vi "Configure Setpoints Range Limits.vi"(7 "Unit Address (1)":u8=1, 8 "error in (no error)":errorcluster, 9 "Range Limit Value (0)":i32, 10 "Limit Type (False)":bool, 11 "VISA resource name":refnum<visa-resource-name>) -> (0 "error out":errorcluster, 3 "VISA resource name out":refnum<visa-resource-name>)   [LabVIEW 2014, in "Eurotherm 35xx Series.lvlib"]
doc: "This VI sets the Range limits of Setpoints.\n\nWarning: This VI uses Controller Configuration Mode, this interrupts working process (device will not control).\nIt is recommended that the device should be disconnected from any active process."
uses:
  <instrlib>/Eurotherm 35xx Series/Eurotherm 35xx Series.lvlib
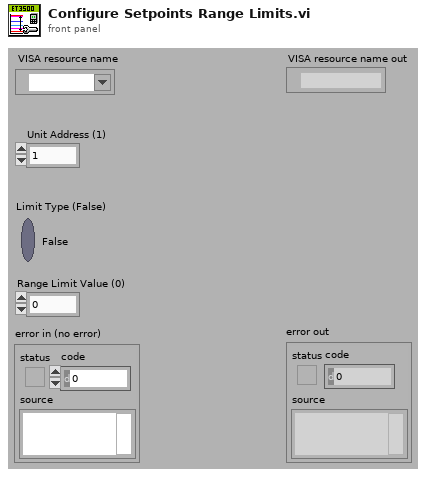
[diagram p1: front panel]
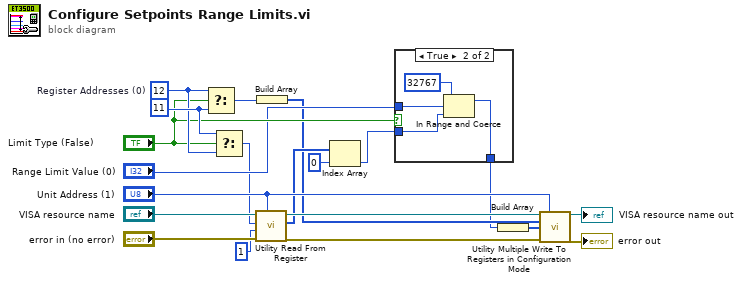
[diagram p0: block diagram]
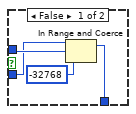
[diagram p2: hidden frame]
diagram:
  w12 = 11 ("Register Addresses (0)")
  w11 = 12  # Register Addresses (0)
  n1 = Select(t=w11, s="Limit Type (False)", f=w12) -> (s? t:f=w4:i32)
  n2 = Select(t=w12, s="Limit Type (False)", f=w11) -> (s? t:f=w5:i32)
  n3 = call <instrlib>:"Utility Read From Register.vi"("Unit Address (1)"="Unit Address (1)", "error in (no error)"="error in (no error)", "Num Of Reg (1)"=u16 1, "Register Address (0)"=w5, "VISA resource name"="VISA resource name") -> ("error out"=w16:errorcluster, "Data"=w10:i16[], "VISA resource name out"=w17:refnum<visa-resource-name>)  [unwired: 4 in]
  n4 = Build Array(w4) -> (w3:i32[])
  n5 = Index Array(array=w10, index=0) -> (element=w7:i16)
  n6 = case shown="True" "Limit Type (False)" {
    tunnel: w7 -> [w22 w27]
    tunnel: "Range Limit Value (0)" -> [w24 w26]
    tunnel: [w21 w25] -> w1
    frame False {
      n7 = In Range and Coerce(upper limit=w22, x=w24, lower limit=-32768 ("upper limit")) -> (coerced(x)=w21:i32)  [unwired: 1 out]
    }
    frame True {
      n8 = In Range and Coerce(upper limit=32767, x=w26, lower limit=w27) -> (coerced(x)=w25:i32)  [unwired: 1 out]
    }
  }
  n9 = Build Array(w1) -> (w2:i32[])
  n10 = call <instrlib>:"Utility Multiple Write To Registers in Configuration Mode.vi"("VISA resource name"=w17, "Unit Address (1)"="Unit Address (1)", "Registers Addresses (0)"=w3, "Data (0)"=w2, "error in (no error)"=w16) -> ("VISA resource name out"=→"VISA resource name out":refnum<visa-resource-name>, "error out"=→"error out":errorcluster)  [unwired: 9 in]
